vi "Wait For Operation Complete.vi"(8 "error in (no error)":errorcluster, 10 "Maximum Time (10000ms)":u32=10000, 11 "VISA resource name":refnum<visa-resource-name>) -> (0 "error out":errorcluster, 3 "VISA resource name out":refnum<visa-resource-name>)   [LabVIEW 2012, in "Agilent 8000 Series.lvlib"]
doc: "Initiates a waveform acquisition. After you call this VI, the instrument leaves the Idle state and waits for a trigger.\n\n<B>Note:</B> Use this VI only with other low-level VIs. The high-level VIs automatically incorporate this functionality. This VI does not check the instrument status."
uses:
  Agilent 8000 Series.lvlib
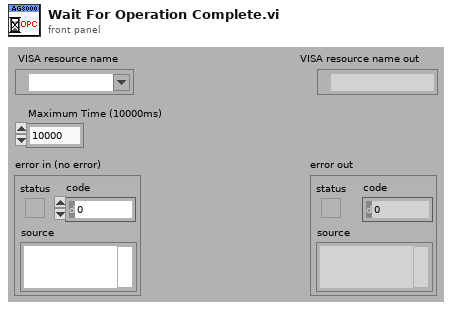
[diagram p1: front panel]
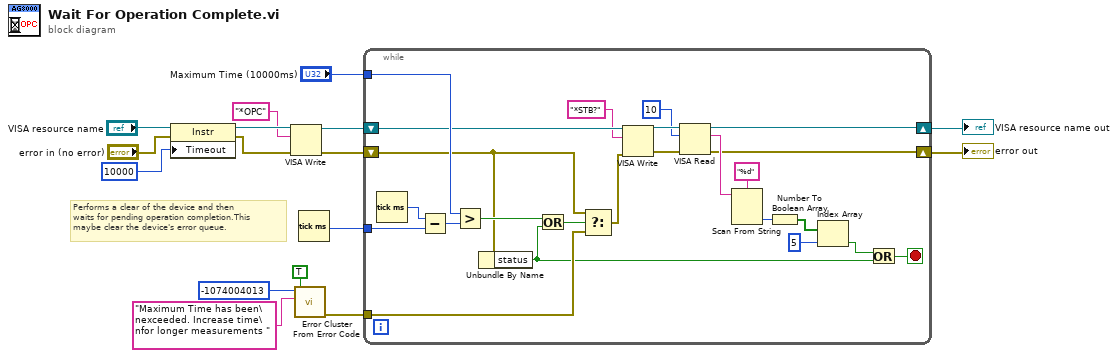
[diagram p0: block diagram]
diagram:
  # "Performs a clear of the device and then \nwaits for pending operation completion.This \nmaybe clear the device's error queue."
  n1 = property class="Instr"(reference="VISA resource name", error in="error in (no error)", "Timeout"=u32 10000 ("General Settings:Timeout Value")) -> (reference out=w3:refnum<visa-resource-name>, error out=w2:errorcluster)
  n2 = VISA Write(VISA resource name=w3, write buffer="*OPC", error in (no error)=w2) -> (VISA resource name out=w5:refnum<visa-resource-name>, error out=w4:errorcluster)  [unwired: 1 out]
  n3 = call <vilib>:"Error Cluster From Error Code.vi"("show call chain? (False)"=TRUE, "error message (\"\")"="Maximum Time has been\nexceeded. Increase time\nfor longer measurements " ("error message (\"\")"), "error code (0)"=-1074004013) -> ("error out"=w12:errorcluster)  [unwired: 6 in]
  n4 = Tick Count (ms)() -> (millisecond timer value=w16:u32)
  n5 = while {
    tunnel: w16 -> [w39]
    tunnel: "Maximum Time (10000ms)" -> [w37]
    tunnel: w12 -> [w34]
    shift-right: [w26] -> w10
    shift-left: w5 -> [w32]
    shift-right: [w23] -> w9
    shift-left: w4 -> [w33]
    stop <- w22 stop-if-true
    n6 = Tick Count (ms)() -> (millisecond timer value=w40:u32)
    n7 = Subtract(x=w40, y=w39) -> (x-y=w38:u32)
    n8 = Greater?(x=w37, y=w38) -> (0:w36:bool)
    n9 = Unbundle By Name(w33) -> ("status"=w17:bool)
    n10 = Or(x=w36, y=w17) -> (x .or. y?=w35:bool)
    n11 = Select(t=w33, s=w35, f=w34) -> (s? t:f=w31:errorcluster)
    n12 = VISA Write(VISA resource name=w32, write buffer="*STB?", error in (no error)=w31) -> (VISA resource name out=w29:refnum<visa-resource-name>, error out=w28:errorcluster)  [unwired: 1 out]
    n13 = VISA Read(VISA resource name=w29, byte count=u32 10, error in (no error)=w28) -> (VISA resource name out=w26:refnum<visa-resource-name>, read buffer=w25:string, error out=w23:errorcluster)  [unwired: 1 out]
    n14 = Scan From String(format string="%d", input string=w25) -> (output 1=w21:i32)  [unwired: 3 in, 3 out]
    n15 = Number To Boolean Array(number=w21) -> (Boolean array=w20:bool[])
    n16 = Index Array(array=w20, index=5) -> (element=w18:bool)
    n17 = Or(x=w18, y=w17) -> (x .or. y?=w22:bool)
  }
  "error out" <- w9
  "VISA resource name out" <- w10
